vi "Bedingte Deaktivierung aendern.vi"() -> ()   [LabVIEW 2020]
uses:
  <vilib>/Utility/file.llb/Read Delimited Spreadsheet (string).vi
  Allgemein/allgemeine Sub-VIs.lvlib
  ConditionalDeactivation/ConditionalDeactivation.lvlib
panel:
  in  "Neue Datei erstellen":bool
  # "1) Button True = erstellt eine neue Datei\n    Button False = liest die ausgewählte Datei ein\n\n2) Play drücken"
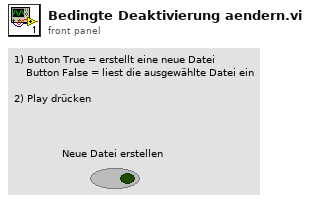
[diagram p1: front panel]
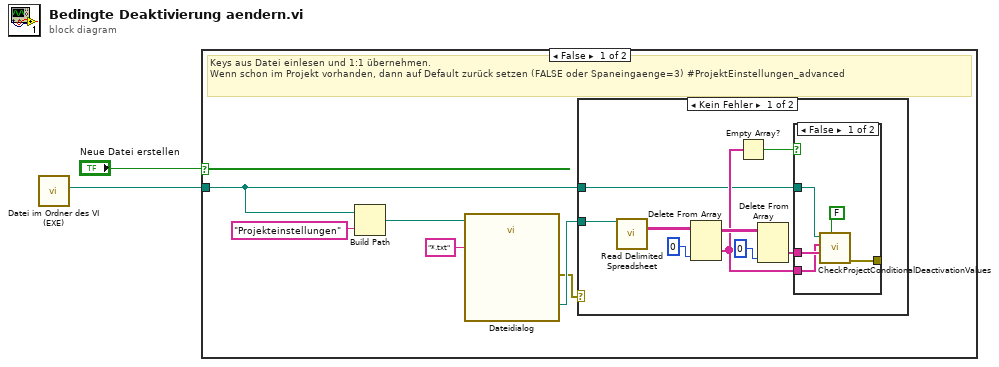
[diagram p0: block diagram]
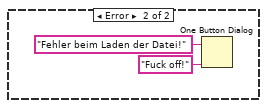
[diagram p3: hidden frame]
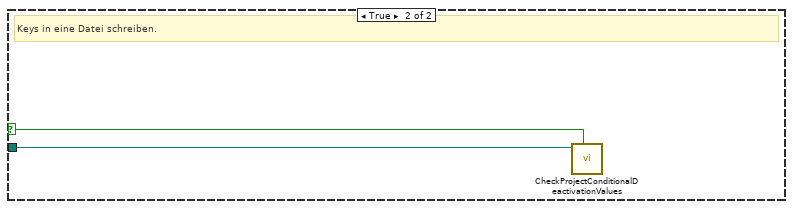
[diagram p4: hidden frame]
diagram:
  n1 = call "Datei im Ordner des VI (EXE).vi"() -> ("Ordner des Haupt-VIs"=w1:path)  [unwired: 9 in, 2 out]
  n2 = case shown="False" "Neue Datei erstellen" {
    selector: "Neue Datei erstellen" -> [_ w25]
    tunnel: w1 -> [w7 w26]
    frame False {
      # "Keys aus Datei einlesen und 1:1 übernehmen.\nWenn schon im Projekt vorhanden, dann auf Default zurück setzen (FALSE oder Spaneingaenge=3) #ProjektEinstellungen_advanced"
      n3 = Build Path(base path=w7, name or relative path="Projekteinstellungen") -> (appended path=w5:path)
      n4 = call "Dateidialog"("start path"=w5, "pattern (all files)"="*.txt") -> ("selected path"=w8:path, "error out"=w4:errorcluster)  [unwired: 10 in, 2 out]
      n5 = case shown="Kein Fehler" w4 {
        tunnel: w8 -> [w10 _]
        tunnel: w7 -> [w9 _]
        frame No Error {
          n6 = call-poly <vilib>:"Read Delimited Spreadsheet.vi"("file path (dialog if empty)"=w10) -> ("all rows"=w17:string[][])  [unwired: 9 in, 5 out]
          n7 = Delete From Array(array=w17, index (col)=0 ("Deaktivierter Index (Spalte)")) -> (deleted portion=w12:string[], array with subset deleted=w15:string[][])  [unwired: 2 in]
          n8 = Empty Array?(array=w12) -> (empty?=w11:bool)
          n9 = Delete From Array(array=w15, index (col)=0 ("Deaktivierter Index (Spalte)")) -> (deleted portion=w13:string[])  [unwired: 2 in, 1 out]
          n10 = case shown="False" w11 {
            tunnel: w13 -> [w22 _]
            tunnel: w9 -> [w21 _]
            tunnel: [w20 _] -> _
            tunnel: w12 -> [w19 _]
            frame False {
              n11 = call "CheckProjectConditionalDeactivationValues.vi"("Datei erstellen"=FALSE, "Value aus Datei"=w22, "Key aus Datei"=w19, "Project Path"=w21) -> ("Fehler (Ausgang)"=w20:errorcluster)  [unwired: 6 in, 1 out]
            }
            frame True {
            }
          }
        }
        frame Error {
          n12 = One Button Dialog(message="Fehler beim Laden der Datei!" ("Nachricht"), button name ("OK")="Fuck off!" ("Schaltflächentext (\"OK\")")) -> ()  [unwired: 1 out]
        }
      }
    }
    frame True {
      # "Keys in eine Datei schreiben."
      n13 = call "CheckProjectConditionalDeactivationValues.vi"("Datei erstellen"=w25, "Project Path"=w26) -> ()  [unwired: 8 in, 2 out]
    }
  }
